vi "DriveNetwork.vi"(8 "error in (no error)":errorcluster) -> (0 "error out":errorcluster)   [LabVIEW 2023]
doc: "Network for Drive\n\nInputs:\n -- Error in -- Error cluster -- propagated error input\n\nOutputs:\n -- Error out -- Error cluster -- progated error output"
uses:
  <vilib>/Rock Robotics/Network Tables/NT Write Number.vi
  DriveGlobal.vi
  <vilib>/Rock Robotics/Network Tables/NT Write Boolean.vi
  <vilib>/Rock Robotics/Network Tables/NT Read Boolean.vi
  <vilib>/Rock Robotics/Network Tables/NT Read Number.vi
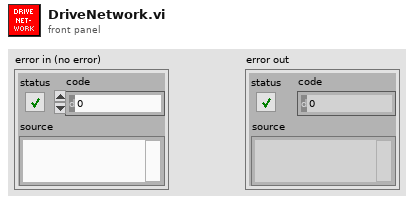
[diagram p1: front panel]
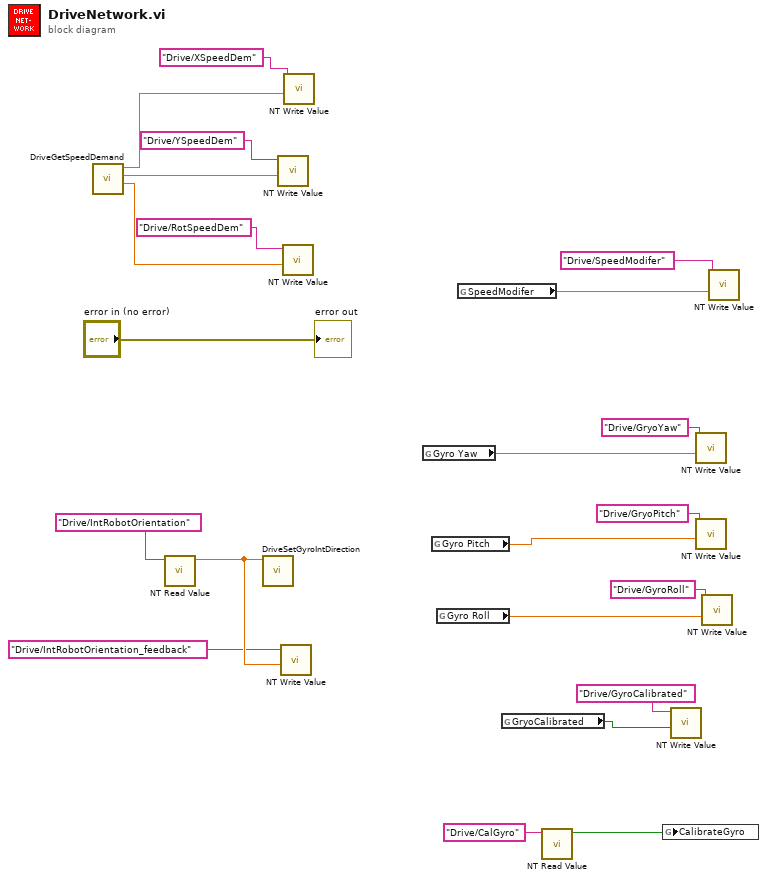
[diagram p0: block diagram]
diagram:
  n1 = call "DriveGetSpeedDemand.vi"() -> ("vOmega"=w4:dbl, "vY"=w20:dbl, "vX"=w21:dbl)  [unwired: 8 in, 1 out]
  n2 = call-poly <vilib>:"NT Read Value.vi"("name"="Drive/IntRobotOrientation") -> ("value"=w2:dbl)  [unwired: 8 in, 2 out]
  n3 = call "DriveSetGyroIntDirection.vi"("GyroIntDirection"=w2) -> ()  [unwired: 11 in]
  n4 = call-poly <vilib>:"NT Write Value.vi"("value"=w20, "name"="Drive/YSpeedDem") -> ()  [unwired: 9 in, 1 out]
  n5 = call-poly <vilib>:"NT Write Value.vi"("value"=w2, "name"="Drive/IntRobotOrientation_feedback") -> ()  [unwired: 9 in, 1 out]
  n6 = call-poly <vilib>:"NT Write Value.vi"("value"=w4, "name"="Drive/RotSpeedDem") -> ()  [unwired: 9 in, 1 out]
  n7 = call-poly <vilib>:"NT Write Value.vi"("value"=w21, "name"="Drive/XSpeedDem") -> ()  [unwired: 9 in, 1 out]
  n8 = global read "DriveGlobal.vi" "Gyro Yaw"() -> (w14:dbl)
  n9 = global read "DriveGlobal.vi" "Gyro Pitch"() -> (w15:dbl)
  n10 = global read "DriveGlobal.vi" "Gyro Roll"() -> (w16:dbl)
  n11 = global read "DriveGlobal.vi" "SpeedModifer"() -> (w12:dbl)
  n12 = global read "DriveGlobal.vi" "GryoCalibrated"() -> (w6:bool)
  n13 = call-poly <vilib>:"NT Read Value.vi"("name"="Drive/CalGyro") -> ("value"=w7:bool)  [unwired: 8 in, 2 out]
  n14 = global write "DriveGlobal.vi" "CalibrateGyro"(w7) -> ()
  n15 = call-poly <vilib>:"NT Write Value.vi"("value"=w6, "name"="Drive/GyroCalibrated") -> ()  [unwired: 9 in, 1 out]
  n16 = call-poly <vilib>:"NT Write Value.vi"("value"=w14, "name"="Drive/GryoYaw") -> ()  [unwired: 9 in, 1 out]
  n17 = call-poly <vilib>:"NT Write Value.vi"("value"=w15, "name"="Drive/GryoPitch") -> ()  [unwired: 9 in, 1 out]
  n18 = call-poly <vilib>:"NT Write Value.vi"("value"=w16, "name"="Drive/GyroRoll") -> ()  [unwired: 9 in, 1 out]
  n19 = call-poly <vilib>:"NT Write Value.vi"("value"=w12, "name"="Drive/SpeedModifer") -> ()  [unwired: 9 in, 1 out]
  "error out" <- "error in (no error)"
